vi "Kalman Calculation.vi"(6 "R":T1=[[0.1, 0.0, 0.0], [0.0, 0.1, 0.0], [0.0, 0.0, 0.1]], 7 "Use Observation":bool=TRUE, 8 "intervalo":dbl=1.0, 9 "Pk-1|k-1":T1, 10 "x_k-1|k-1":T1=[[0.0, 0.0, 0.0], [0.0, 0.0, 0.0], [0.0, 0.0, 0.0]], 11 "z_k":T1) -> (1 "Conf":dbl, 2 "Pk|k":T1, 3 "x_k|k":T1)   [LabVIEW 2018]
uses:
  <vilib>/Analysis/Matrix/Datatypes/RealMatrix.ctl
  <vilib>/Analysis/_algsub.llb/Real Matrix Norm.vi
  <vilib>/Analysis/Matrix/Numeric/Multiply/Multiply - RM,RM.vi
  <vilib>/Analysis/Matrix/Numeric/Add/Add - RM,RM.vi
  <vilib>/Analysis/Matrix/NI_Matrix.lvlib
  <vilib>/Analysis/NI_AALBase.lvlib
  <vilib>/Analysis/baseanly.llb/Real Inverse Matrix.vi
  <vilib>/Analysis/NI_AALPro.lvlib
panel:
  out "K_k":T1
  out "Inverse Matrix":T1
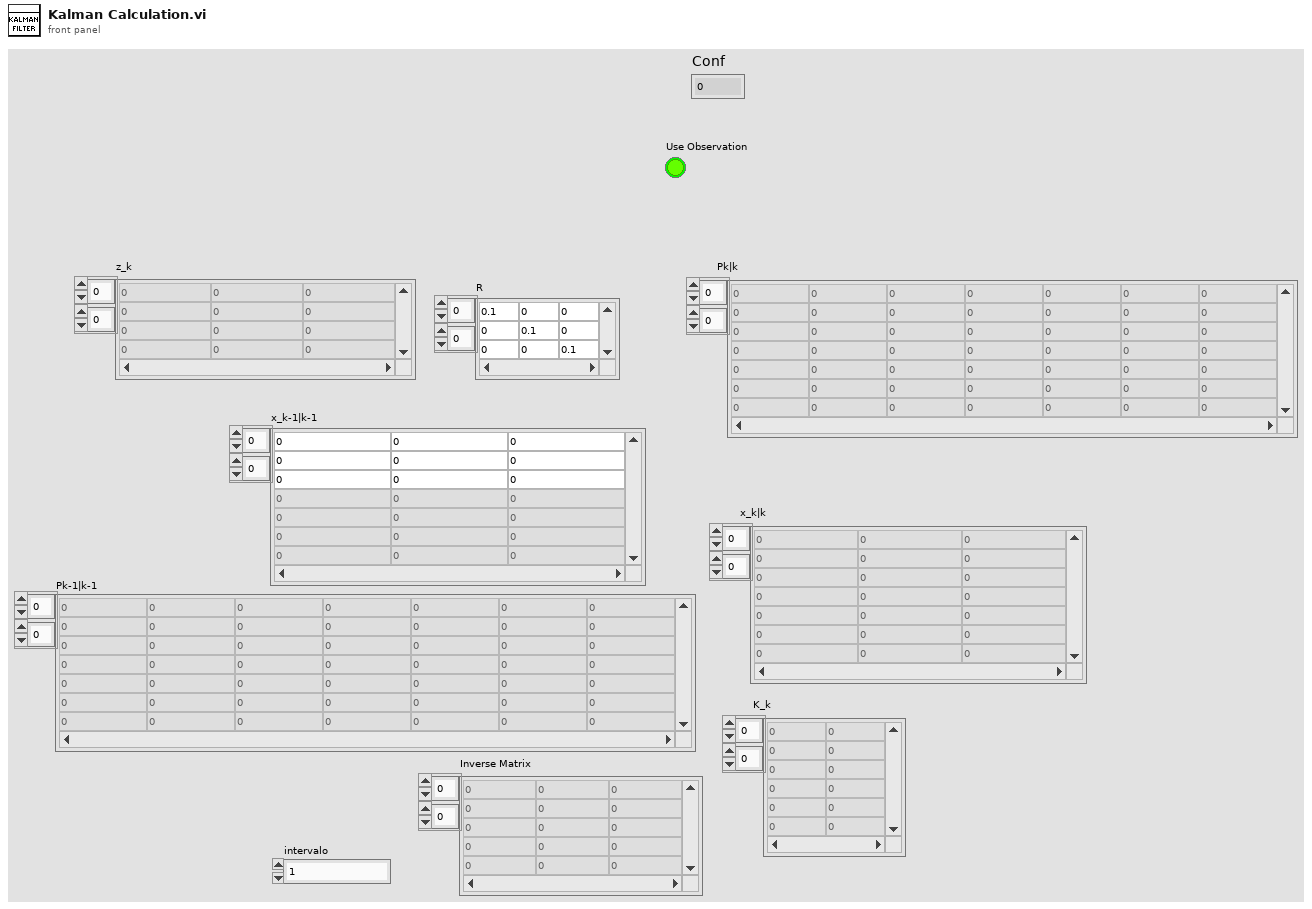
[diagram p1: front panel]
types:
  T1 = typedef "NI_Matrix.lvlib/RealMatrix.ctl" = dbl[][]
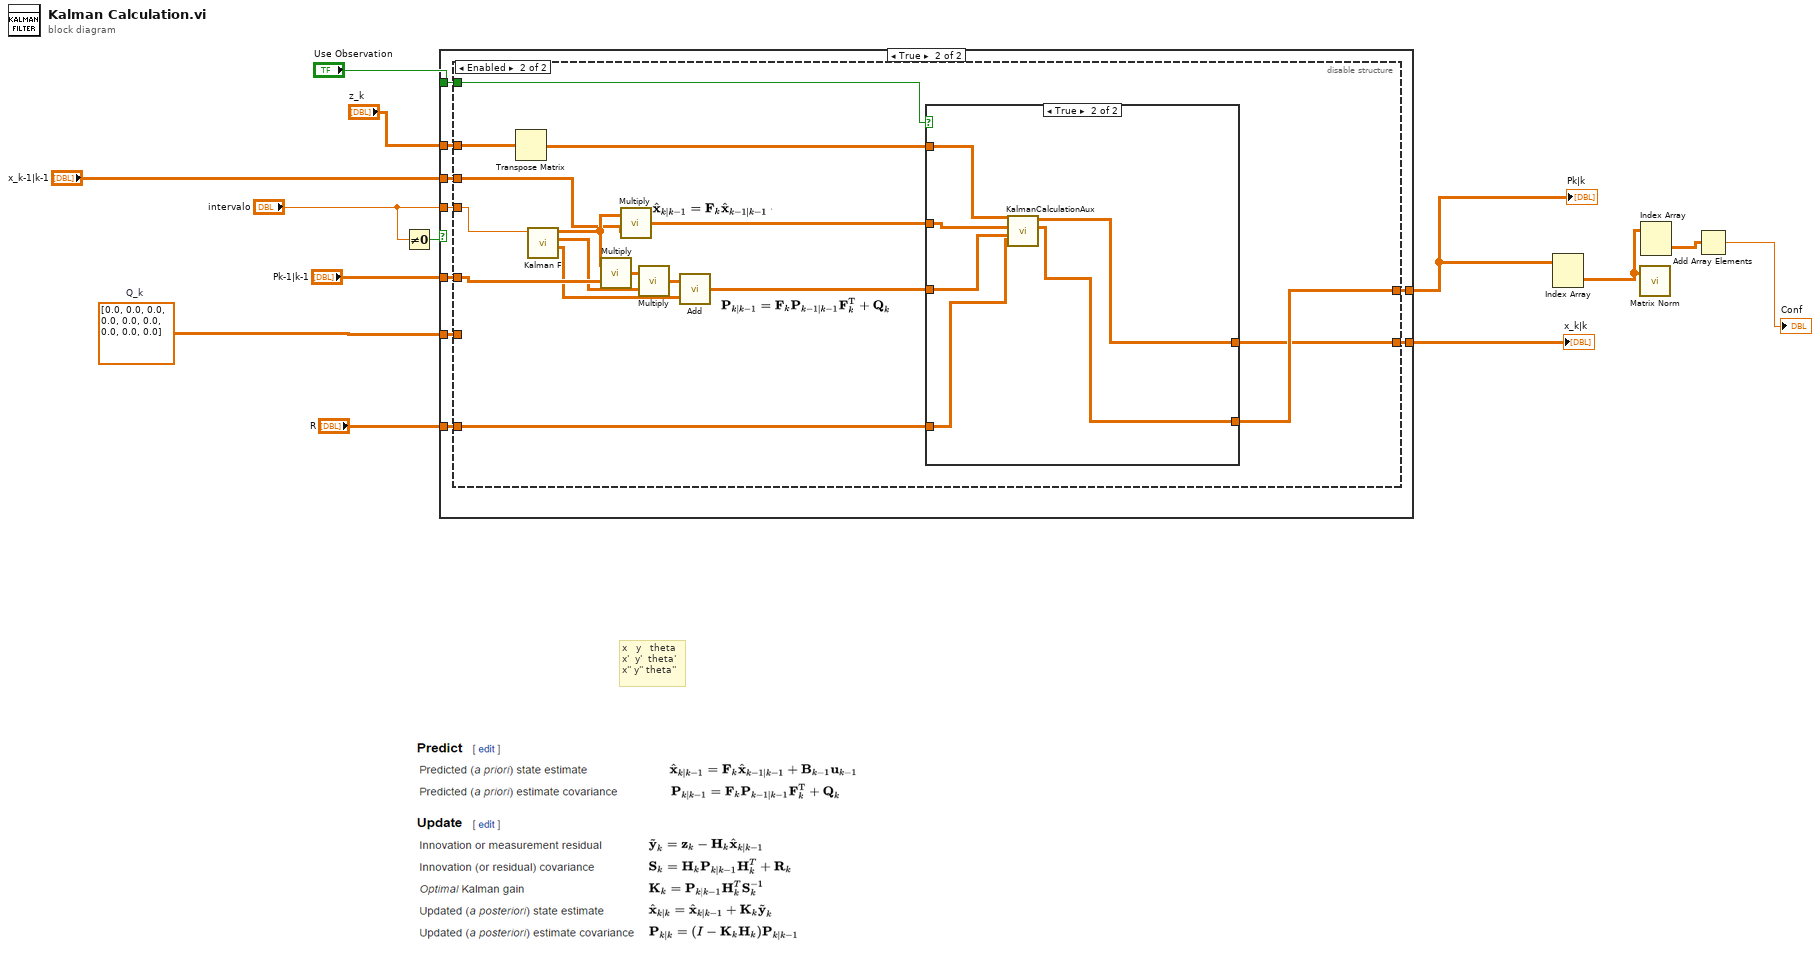
[diagram p0: block diagram]
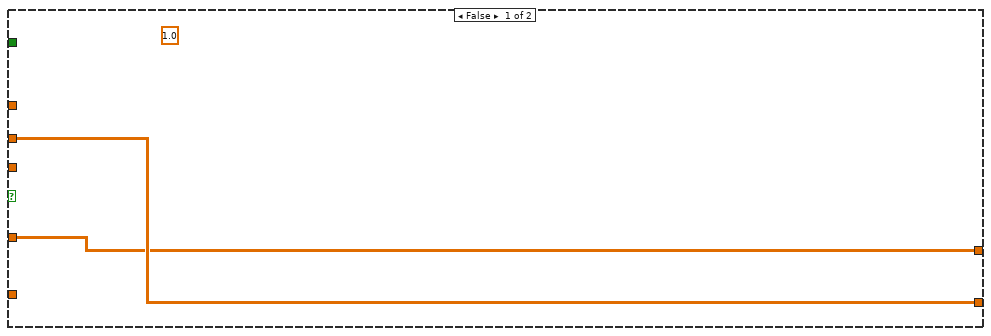
[diagram p2: hidden frame]
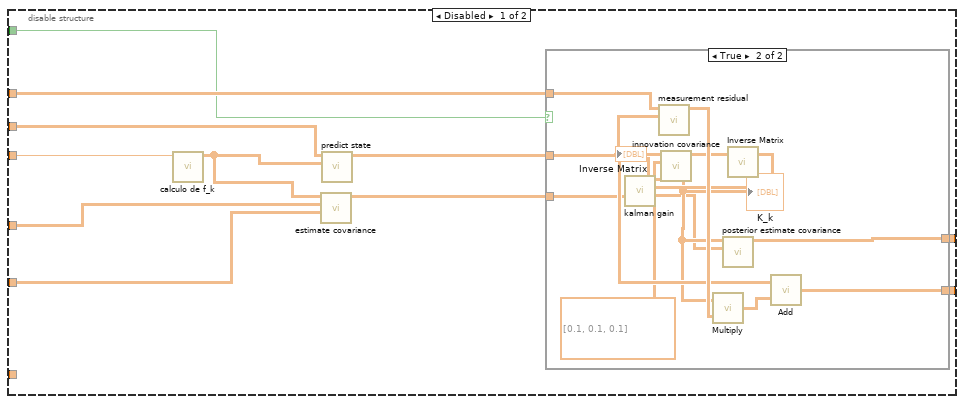
[diagram p3: hidden frame]
diagram:
  w10 = T1 [[0.0, 0.0, 0.0], [0.0, 0.0, 0.0], [0.0, 0.0, 0.0]]  # Q_k
  # "x   y   theta\nx'  y'  theta'\nx'' y'' theta''"
  n1 = Not Equal To 0?(x="intervalo") -> (x != 0?=w11:bool)
  n2 = case shown="True" w11 {
    tunnel: "intervalo" -> [_ w24]
    tunnel: [w15 w23] -> w3
    tunnel: "Pk-1|k-1" -> [w14 w22]
    tunnel: "x_k-1|k-1" -> [w15 w20]
    tunnel: [w14 w21] -> w12
    tunnel: w10 -> [_ w19]
    tunnel: "z_k" -> [_ w18]
    tunnel: "Use Observation" -> [_ w17]
    tunnel: "R" -> [_ w16]
    frame False {
      (unwired) 1.0 ("intervalo")
    }
    frame True {
      n3 = disable-structure shown="Enabled" {
        disable-tunnel: w24 -> [w35 w50]
        disable-tunnel: [w32 w55] -> w23
        disable-tunnel: w22 -> [w31 w64]
        disable-tunnel: [w30 w56] -> w21
        disable-tunnel: w20 -> [w29 w53]
        disable-tunnel: w19 -> [w27 _]
        disable-tunnel: w18 -> [w26 w59]
        disable-tunnel: w17 -> [w25 w51]
        disable-tunnel: w16 -> [_ w52]
        frame Disabled {
          n4 = call "calculo de f_k.vi"("iteração"=w35) -> ("F_k"=w28:T1)  [unwired: 10 in]
          n5 = call "estimate covariance.vi"("Q_k"=w27, "Pk-1|k-1"=w31, "F_k"=w28) -> ("Pk|k-1"=w33:T1)  [unwired: 8 in]
          n6 = call "predict state.vi"("F_k"=w28, "x_k-1|k-1"=w29) -> ("x_k|k-1"=w34:T1)  [unwired: 9 in]
          n7 = case shown="True" w25 {
            tunnel: [w37 w47] -> w32
            tunnel: w34 -> [w37 w45]
            tunnel: [w36 w42] -> w30
            tunnel: w33 -> [w36 w40]
            tunnel: w26 -> [_ w39]
            frame False {
            }
            frame True {
              n8 = call "measurement residual.vi"("x_k|k-1"=w45, "z_k"=w39) -> ("y~_k"=w46:T1)  [unwired: 9 in]
              n9 = call "innovation covariance.vi"("R"=T1 [[0.1, 0.1, 0.1]], "Pk|k-1"=w40) -> ("S_k"=w44:T1)  [unwired: 8 in, 1 out]
              n10 = call-poly <vilib>:"Inverse Matrix.vi"("Input Matrix"=w44) -> ("Inverse Matrix"=w43:T1)  [unwired: 1 in, 1 out]
              "Inverse Matrix" <- w43
              n11 = call "kalman gain.vi"("Pk|k-1"=w40, "S^-1"=w43) -> ("K_k"=w41:T1)  [unwired: 9 in]
              "K_k" <- w41
              n12 = call-poly <vilib>:"Multiply.vi"("Real Matrix B"=w46, "Real Matrix A"=w41) -> ("A * B"=w48:T1)
              n13 = call "posterior estimate covariance.vi"("Pk|k-1"=w40, "K_k"=w41) -> ("Pk|k"=w42:T1)  [unwired: 9 in]
              n14 = call-poly <vilib>:"Add.vi"("Real Matrix B"=w48, "Real Matrix A"=w45) -> ("A + B"=w47:T1)
            }
          }
        }
        frame Enabled {
          n15 = Transpose Matrix(1:w59) -> (0:w58:T1)
          n16 = call "Kalman F.vi"("intervalo"=w50) -> ("Q"=w60:T1, "F'"=w62:T1, "F"=w54:T1)  [unwired: 8 in]
          n17 = call-poly <vilib>:"Multiply.vi"("Real Matrix B"=w64, "Real Matrix A"=w54) -> ("A * B"=w63:T1)
          n18 = call-poly <vilib>:"Multiply.vi"("Real Matrix B"=w53, "Real Matrix A"=w54) -> ("A * B"=w49:T1)
          n19 = call-poly <vilib>:"Multiply.vi"("Real Matrix B"=w62, "Real Matrix A"=w63) -> ("A * B"=w61:T1)
          n20 = call-poly <vilib>:"Add.vi"("Real Matrix B"=w60, "Real Matrix A"=w61) -> ("A + B"=w57:T1)
          n21 = case shown="True" w51 {
            tunnel: w58 -> [_ w72]
            tunnel: w49 -> [w66 w67]
            tunnel: w57 -> [w65 w71]
            tunnel: [w65 w68] -> w56
            tunnel: [w66 w69] -> w55
            tunnel: w52 -> [_ w70]
            frame False {
            }
            frame True {
              n22 = call "KalmanCalculationAux.vi"("R"=w70, "A + B in"=w71, "A + B 3"=w67, "z_k"=w72) -> ("A - B"=w68:T1, "A + B out"=w69:T1)  [unwired: 6 in]
            }
          }
        }
      }
    }
  }
  "Pk|k" <- w12
  "x_k|k" <- w3
  n23 = Index Array(array=w12) -> (element=w6:T1)  [unwired: 2 in]
  n24 = call-poly <vilib>:"Matrix Norm.vi"("Input Matrix"=w6) -> ()  [unwired: 1 in, 2 out]
  n25 = Index Array(array=w6) -> (element=w5:T1)  [unwired: 2 in]
  n26 = Add Array Elements(numeric array=w5) -> (sum=→"Conf":dbl)
